vi "speedAquire.vi"(8 "error in (no error)":errorcluster, 11 "VISA resource name":refnum<visa-resource-name>="ASRL6::INSTR") -> (0 "error out (no error)":errorcluster, 1 "FREQUENCY":string, 2 "PWM":string, 3 "KPH/MPH":string, 5 "SPEED":dbl(knob) scale=0.0..25.5)   [LabVIEW 2018]
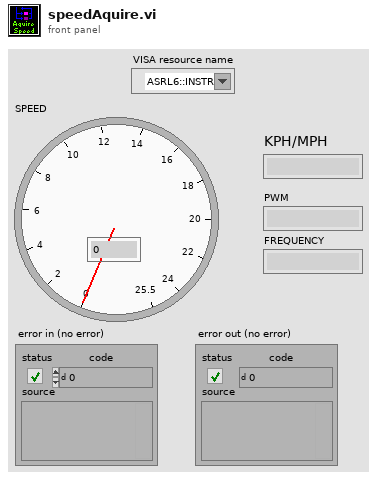
[diagram p1: front panel]
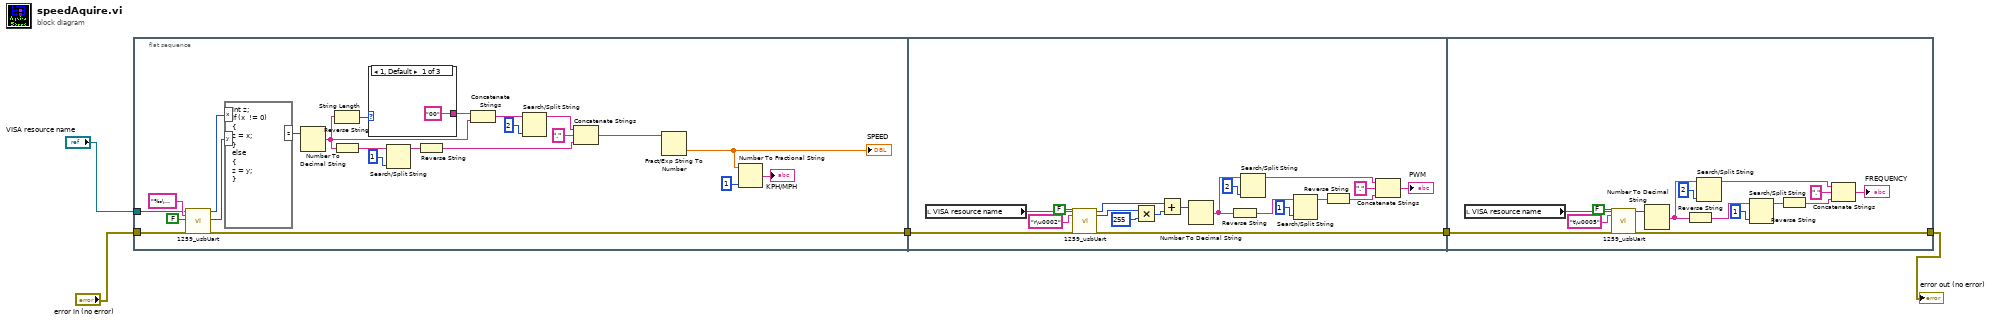
[diagram p0: block diagram]
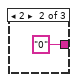
[diagram p2: hidden frame]
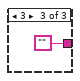
[diagram p3: hidden frame]
diagram:
  n1 = flat-sequence {
    tunnel: "VISA resource name" -> [w18]
    tunnel: "error in (no error)" -> [w13]
    tunnel: [w12] -> w3
    tunnel: w3 -> [w34]
    tunnel: [w33] -> w2
    tunnel: w2 -> [w53]
    tunnel: [w52] -> w1
    frame #0 {
      n2 = call "1259_usbUart.vi"("VISA resource name"=w18, "write buffer"="‰\u0004", "sdFeature"=FALSE, "error in (no error)"=w13) -> ("number[0]"=w27:u32, "number[2]"=w10:u32, "error out"=w12:errorcluster)  [unwired: 13 out]
      n3 = formula code="int z;\nif (x  != 0)\n{\nz = x;\n}\nelse\n{\nz = y;\n}"("x"=w27, "y"=w10) -> ("z"=w28:i32)
      n4 = Number To Decimal String(number=w28) -> (decimal integer string=w15:string)  [unwired: 1 in]
      n5 = String Length(string=w15) -> (length=w17:i32)
      n6 = Reverse String(1:w15) -> (0:w26:string)
      n7 = case shown="1, Default" w17 {
        tunnel: ["00" "0" ""] -> w16
        frame 1, Default {
        }
        frame 2 {
        }
        frame 3 {
        }
      }
      n8 = Search/Split String(string=w26, offset (0)=1) -> (substring before match=w25:string)  [unwired: 1 in, 2 out]
      n9 = Reverse String(1:w25) -> (0:w23:string)
      n10 = Concatenate Strings(w16, w15) -> (w14:string)
      n11 = Search/Split String(string=w14, offset (0)=2) -> (substring before match=w24:string)  [unwired: 1 in, 2 out]
      n12 = Concatenate Strings(w24, "." ("string"), w23) -> (w11:string)
      n13 = Fract/Exp String To Number(string=w11) -> (number=w9:dbl)  [unwired: 3 in, 1 out]
      "SPEED" <- w9
      n14 = Number To Fractional String(number=w9, precision (6)=i16 1) -> (F-format string=→"KPH/MPH":string)  [unwired: 2 in]
    }
    frame #1 {
      n15 = local read "VISA resource name"() -> (w50:refnum<visa-resource-name>)
      n16 = call "1259_usbUart.vi"("VISA resource name"=w50, "write buffer"="r\u0002", "sdFeature"=FALSE, "error in (no error)"=w34) -> ("number[0]"=w45:u32, "number[1]"=w48:u32, "error out"=w33:errorcluster)  [unwired: 13 out]
      n17 = Multiply(x=w48, y=u32 255) -> (x*y=w46:u32)
      n18 = Add(x=w45, y=w46) -> (x+y=w35:u32)
      n19 = Number To Decimal String(number=w35) -> (decimal integer string=w40:string)  [unwired: 1 in]
      n20 = Reverse String(1:w40) -> (0:w43:string)
      n21 = Search/Split String(string=w40, offset (0)=2) -> (substring before match=w37:string)  [unwired: 1 in, 2 out]
      n22 = Search/Split String(string=w43, offset (0)=1) -> (substring before match=w39:string)  [unwired: 1 in, 2 out]
      n23 = Reverse String(1:w39) -> (0:w38:string)
      n24 = Concatenate Strings(w37, "." ("string"), w38) -> (→"PWM":string)
    }
    frame #2 {
      n25 = local read "VISA resource name"() -> (w64:refnum<visa-resource-name>)
      n26 = call "1259_usbUart.vi"("VISA resource name"=w64, "write buffer"="t\u0005", "sdFeature"=FALSE, "error in (no error)"=w53) -> ("number[0]"=w54:u32, "error out"=w52:errorcluster)  [unwired: 14 out]
      n27 = Number To Decimal String(number=w54) -> (decimal integer string=w59:string)  [unwired: 1 in]
      n28 = Reverse String(1:w59) -> (0:w62:string)
      n29 = Search/Split String(string=w59, offset (0)=2) -> (substring before match=w56:string)  [unwired: 1 in, 2 out]
      n30 = Search/Split String(string=w62, offset (0)=1) -> (substring before match=w58:string)  [unwired: 1 in, 2 out]
      n31 = Reverse String(1:w58) -> (0:w57:string)
      n32 = Concatenate Strings(w56, "." ("string"), w57) -> (→"FREQUENCY":string)
    }
  }
  "error out (no error)" <- w1
